vi "Query PRACH Modulation Limit Check Results.vi"(0 "VISA resource name":refnum<visa-resource-name>, 5 "Instance (1)":T1=1, 7 "Result Type (Current)":i32(ring) items=["Current", "Average"], 11 "error in (no error)":errorcluster) -> (4 "VISA resource name out":refnum<visa-resource-name>, 6 "Reliability":i32, 8 "Out Of Tolerance":i32, 10 "Limit Check Results":i32[](array[numeric]), 15 "error out":errorcluster)   [LabVIEW 2020, in "Rohde&Schwarz CMWXP NR FR1 Measurement.lvlib"]
doc: "Returns the limit check results for the single value modulation results.\n\nAttributes:\nRSCMWXPNRFR1M_ATTR_QUERY_PRACH_MODULATION_CURRENT_LIMIT_CHECK_RESULTS\nRSCMWXPNRFR1M_ATTR_QUERY_PRACH_MODULATION_AVERAGE_LIMIT_CHECK_RESULTS\n\nRemote-control commands:\nCALCulate:NRSub:MEAS<i>:PRACh:MODulation:CURRent?\nCALCulate:NRSub:MEAS<i>:PRACh:MODulation:AVERage?"
uses:
  <instrlib>/Rohde&Schwarz CMWXP NR FR1 Measurement/Rohde&Schwarz CMWXP NR FR1 Measurement.lvlib
  <instrlib>/Rohde&Schwarz CMWXP NR FR1 Measurement/Private/_Instance.ctl
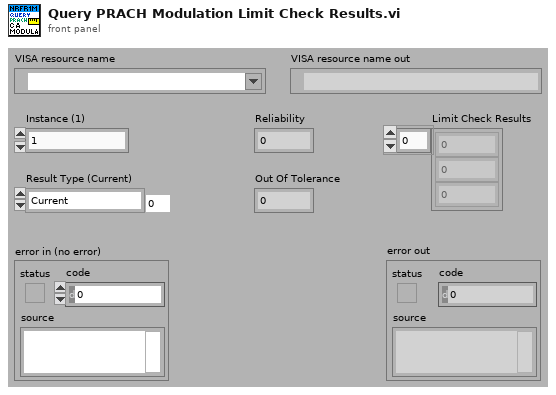
[diagram p1: front panel]
types:
  T1 = typedef "Rohde&Schwarz CMWXP NR FR1 Measurement.lvlib/_Instance.ctl" = i32
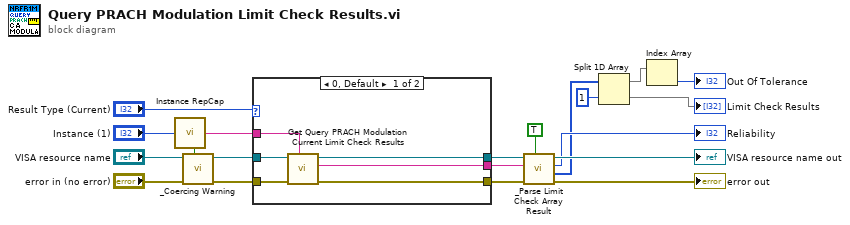
[diagram p0: block diagram]
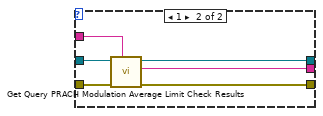
[diagram p2: hidden frame]
diagram:
  n1 = call <instrlib>:"Instance RepCap.vi"("Instance In"="Instance (1)") -> ("In Range?"=w20:bool, "RepCap Identifier Out"=w14:string)  [unwired: 1 in]
  n2 = call <instrlib>:"_Coercing Warning.vi"("In Range?"=w20, "error in (no error)"="error in (no error)", "VISA resource name"="VISA resource name") -> ("error out"=w18:errorcluster, "VISA resource name out"=w15:refnum<visa-resource-name>)  [unwired: 7 in]
  n3 = case shown="0, Default" "Result Type (Current)" {
    tunnel: w15 -> [w26 w32]
    tunnel: w18 -> [w25 w31]
    tunnel: w14 -> [w24 w30]
    tunnel: [w23 w27] -> w11
    tunnel: [w22 w29] -> w9
    tunnel: [w21 w28] -> w10
    frame 0, Default {
      n4 = call "Get Query PRACH Modulation Current Limit Check Results"("Repeated Capabilities"=w24, "error in (no error)"=w25, "instrument handle"=w26) -> ("error out"=w23:errorcluster, "Query PRACH Modulation Current Limit Check Results"=w21:string, "instrument handle out"=w22:refnum<visa-resource-name>)  [unwired: 6 in]
    }
    frame 1 {
      n5 = call "Get Query PRACH Modulation Average Limit Check Results"("Repeated Capabilities"=w30, "error in (no error)"=w31, "instrument handle"=w32) -> ("error out"=w27:errorcluster, "Query PRACH Modulation Average Limit Check Results"=w28:string, "instrument handle out"=w29:refnum<visa-resource-name>)  [unwired: 6 in]
    }
  }
  n6 = call <instrlib>:"_Parse Limit Check Array Result.vi"("error in (no error)"=w11, "Input String"=w10, "VISA resource name"=w9, "Out of tolerance? (F)"=TRUE) -> ("error out"=→"error out":errorcluster, "Results"=w5:i32[], "Reliability"=→"Reliability":i32, "VISA resource name out"=→"VISA resource name out":refnum<visa-resource-name>)  [unwired: 2 in, 1 out]
  n7 = Split 1D Array(array=w5, index=1) -> (first subarray=w2:i32[], second subarray=→"Limit Check Results":i32[])
  n8 = Index Array(array=w2) -> (element=→"Out Of Tolerance":i32)  [unwired: 1 in]
